vi "Write Interlock_Enable.vi"(8 "error in":errorcluster, 10 "INTLK_Enable":bool, 11 "57XX in":refnum<class "57XX.lvclass">) -> (0 "error out":errorcluster, 3 "57XX out":refnum<class "57XX.lvclass">)   [LabVIEW 2019, in "57XX.lvlib" / "57XX.lvclass"]
uses:
  Library/57XX.lvclass
  C:/Users/Public/Documents/Development/builds/Engine/Monitored Actor.lvlibp/Monitored Actor/Monitored Actor/Monitored Actor.lvclass
  builds/Engine/Monitored Actor.lvlibp/Monitored Actor/Monitored Actor/Read Actor Label.vi
  builds/Instruments/PowerSupply.lvlibp/Library/PowerSupply.lvclass
  <vilib>/ErrorRing/Error Ring.xnode
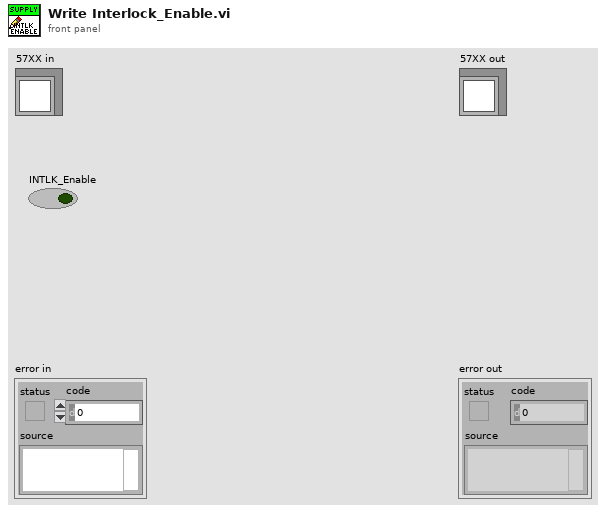
[diagram p1: front panel]
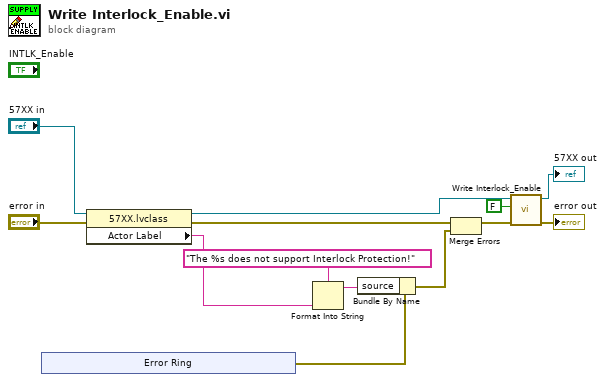
[diagram p0: block diagram]
diagram:
  n1 = xnode "Error Ring"() -> ("error out"=w6:errorcluster)
  n2 = property class="57XX.lvclass"(reference="57XX in", error in="error in") -> (reference out=w8:refnum<class "57XX.lvclass">, error out=w7:errorcluster, "Actor Label"=w3:string)
  n3 = Format Into String(format string="The %s does not support Interlock Protection!", w3) -> (resulting string=w5:string)  [unwired: 2 in, 1 out]
  n4 = Bundle By Name(cluster=w6, "source"=w5) -> (w4:errorcluster)
  n5 = Merge Errors(w7, w4) -> (w11:errorcluster)
  n6 = call-parent "Write Interlock_Enable.vi"("error in"=w11, "INTLK_Enable"=FALSE, "PowerSupply in"=w8) -> ("error out"=→"error out":errorcluster, "PowerSupply out"=→"57XX out":refnum<class "57XX.lvclass">)  [unwired: 7 in]
